vi "Constructor.vi"(8 "error in (no error)":errorcluster) -> (0 "error out":errorcluster, 3 "CollectionByRef out":refnum<class "CollectionByRef.lvclass">)   [LabVIEW 2021, in "Collection.lvlib" / "CollectionByRef.lvclass"]
uses:
  CollectionByRef.lvclass
  CollectionByValue/CollectionByValue.lvclass
  CollectionByRef.lvclass/CollectionByRef.ctl
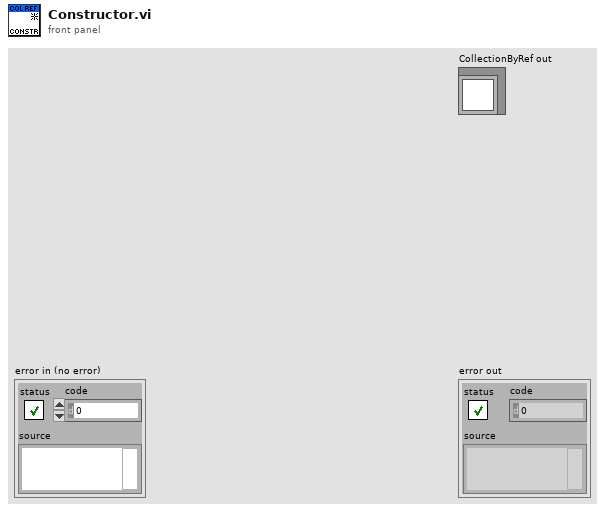
[diagram p1: front panel]
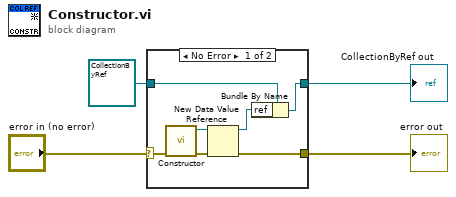
[diagram p0: block diagram]
diagram:
  n1 = case shown="No Error" "error in (no error)" {
    selector: "error in (no error)" -> [w9 w13]
    tunnel: [w11 w13] -> w3
    tunnel: [w7 w12] -> w2
    tunnel: refnum<class "CollectionByRef.lvclass"> refnum ("CollectionByRef out") -> [w5 w12]
    frame No Error {
      n2 = call "Constructor.vi"("error in (no error)"=w9) -> ("error out"=w8:errorcluster, "Collection out"=w10:refnum<class "CollectionByValue.lvclass">)  [unwired: 9 in]
      n3 = New Data Value Reference(data value=w10, error in=w8) -> (data value reference=w6:refnum<data-value>, error out=w11:errorcluster)
      n4 = Bundle By Name(cluster=w5, "ref"=w6) -> (w7:refnum<class "CollectionByRef.lvclass">)
    }
    frame Error {
    }
  }
  "error out" <- w3
  "CollectionByRef out" <- w2
